vi "Read configuration.vi"(8 "error in":errorcluster, 11 "NISE_CEF_serializable node folder in":refnum<class "NISE_CEF_serializable node folder.lvclass">) -> (0 "error out":errorcluster, 2 "configuration":refnum<class "NISE_CEF_serializable configuration.lvclass">, 3 "NISE_CEF_serializable node folder out":refnum<class "NISE_CEF_serializable node folder.lvclass">)   [LabVIEW 2013, in "NISE_CEF_serializable node folder.lvclass"]
uses:
  NISE_CEF_serializable node folder.lvclass
  serializable configuration/NISE_CEF_serializable configuration.lvclass
  NISE_CEF_serializable node folder.lvclass/NISE_CEF_serializable node folder.ctl
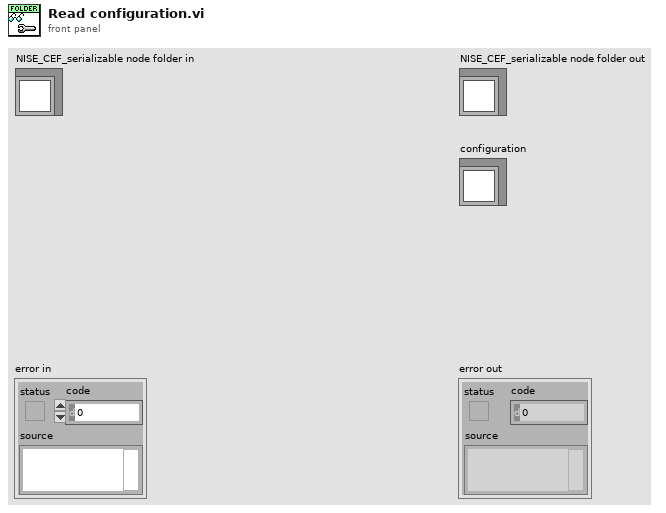
[diagram p1: front panel]
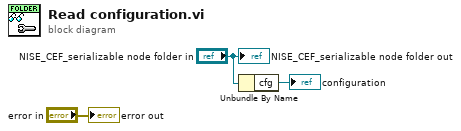
[diagram p0: block diagram]
diagram:
  n1 = Unbundle By Name("NISE_CEF_serializable node folder in") -> ("cfg"=→"configuration":refnum<class "NISE_CEF_serializable node folder configuration.lvclass">)
  "error out" <- "error in"
  "NISE_CEF_serializable node folder out" <- "NISE_CEF_serializable node folder in"
